vi "string of n items.vi"(1 "string":string, 2 "Numeric":dbl) -> (0 "String":string)   [LabVIEW 2017]
doc: "This creates a string of \"n\" items of object \"m\", where n and m are the two inputs."
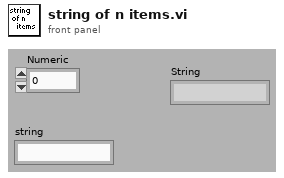
[diagram p1: front panel]
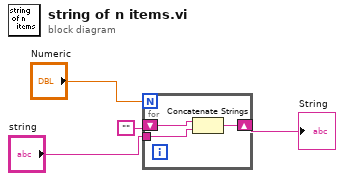
[diagram p0: block diagram]
diagram:
  n1 = for {
    N: "Numeric" -> [_]
    shift-right: [w7] -> w2
    shift-left: "" -> [w6]
    tunnel: "string" -> [w5]
    n2 = Concatenate Strings(w6, w5) -> (w7:string)
  }
  "String" <- w2
